vi "Database_Patient_Info.vi"() -> ()   [LabVIEW 2013, in "Medimatic.lvlib"]
uses:
  Medimatic.lvlib
  Globals/DataPathGlobalVariable.vi
  <userlib>/LVT/SQLite/Core/Insert/SQLite_Insert Table.vi
panel:
  in  "Value Table":string[][](array[string])
  in  "Column":string[](array[string])
  in  "Patien_ID":string="[Patient_ID]_Measurements"
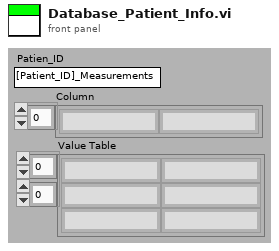
[diagram p1: front panel]
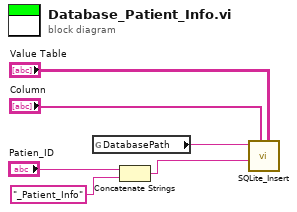
[diagram p0: block diagram]
diagram:
  n1 = global read "DataPathGlobalVariable.vi" "DatabasePath"() -> (w6:string)
  n2 = Concatenate Strings("Patien_ID", "_Patient_Info") -> (w3:string)
  n3 = call-poly <userlib>:"SQLite_Insert.vi"("Value Table"="Value Table", "Column"="Column", "Tabe Name"=w3, "DB Path"=w6) -> ()  [unwired: 3 in, 3 out]
